vi "Fetch Y Trace.vi"(8 "error in (no error)":errorcluster {"code" format="%.0x"}, 9 "array length":i32=1 caption="array length (1)" format="%.0g", 10 "trace name":string="Trace1" caption="trace name (Trace1)", 11 "instrument handle":refnum<k15>) -> (0 "error out":errorcluster {"code" format="%.0x"}, 1 "actual points":i32 format="%.0g", 2 "amplitude":dbl[](array[numeric]), 3 "instrument handle out":refnum<k15>)   [LabVIEW 2009, in "Keysight XSAn.lvlib"]
doc: "This VI returns the trace the spectrum analyzer aquires.\n\nSupported Models: M9290A, N8973B, N8974B, N8975B, N8976B, N9000A, N9000B, N9010A, N9010B, N9020A, N9020B, N9030A, N9030B, N9038A, N9040B, N9041B, SPN9003A, SPN9026A"
uses:
  <instrlib>/Keysight XSAn/Keysight XSAn.lvlib
  AgXSAn.dll
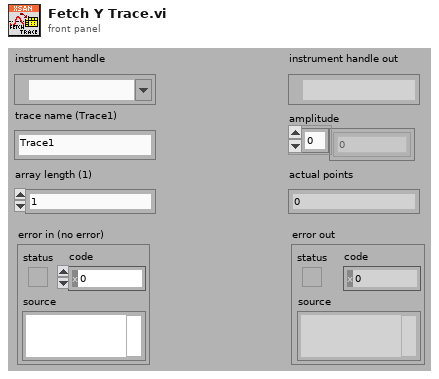
[diagram p1: front panel]
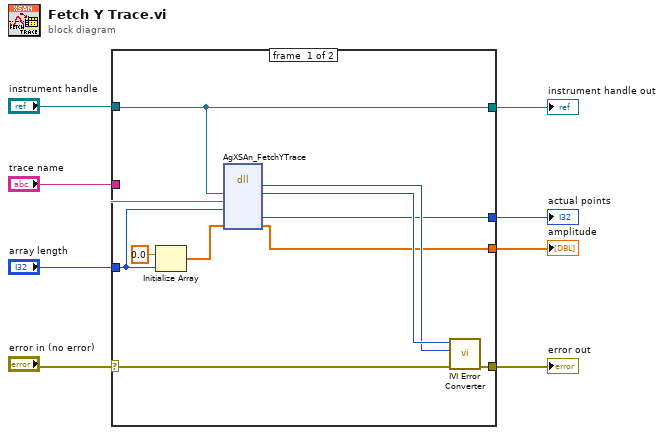
[diagram p0: block diagram]
diagram:
  n1 = case shown="No Error" "error in (no error)" {
    selector: "error in (no error)" -> [w15 w21]
    tunnel: [w16 w21] -> w7
    tunnel: "instrument handle" -> [w11 w20]
    tunnel: "trace name" -> [w13 _]
    tunnel: "array length" -> [w12 _]
    tunnel: [w11 w20] -> w3
    tunnel: [w10 _] -> w2
    tunnel: [w9 _] -> w1
    frame #0 {
      n2 = Initialize Array(0.0, w12) -> (w18:dbl[])
      n3 = dll-call lib="AgXSAn**.dll" fn="AgXSAn_FetchYTrace" ("LabVIEW:IviSpecAn_FetchYTrace")("instrument handle"=w11, "trace name"=w13, "array length"=w12, "amplitude"=w18) -> ("Status"=w14:i32, "instrument handle"=w17:u32, "actual points"=w10:i32, "amplitude"=w9:dbl[])  [unwired: 5 in, 3 out]
      n4 = call <instrlib>:"IVI Error Converter.vi"("error in (no error)"=w15, "IVI error code (0)"=w14, "instrument handle"=w17) -> ("error out"=w16:errorcluster)  [unwired: 7 in, 1 out]
    }
    frame #1 {
    }
  }
  "error out" <- w7
  "instrument handle out" <- w3
  "actual points" <- w2
  "amplitude" <- w1
